vi "Set Focus Slider.vi"(8 "error in (no error)":errorcluster, 10 "Camera Parameter Information":T1, 11 "UI in":refnum<class "UI.lvclass">) -> (0 "error out":errorcluster)   [LabVIEW 2020, in "AR Example.lvlib" / "UI.lvclass"]
uses:
  UI.lvclass
  UI.lvclass/UI.ctl
  <vilib>/Utility/miscctls.llb/LVOutOfRangeActionTypeDef.ctl
  g_ar_toolkit.capture/Stream/Camera Parameter Information.ctl
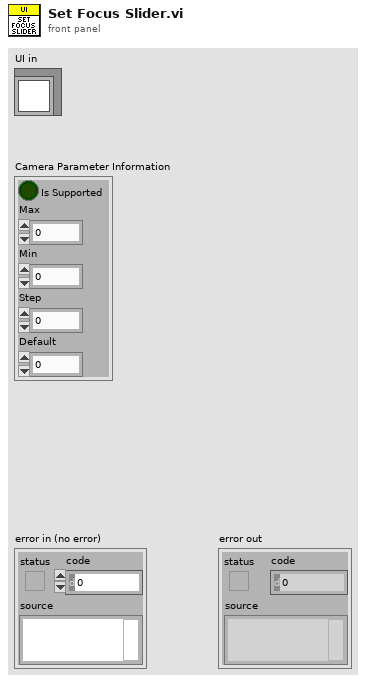
[diagram p1: front panel]
types:
  T1 = typedef "g_ar_toolkit.capture.lvlib/Stream.lvclass/Camera Parameter Information.ctl" = cluster{"Is Supported":bool, "Max":i32, "Min":i32, "Step":i32, "Default":i32}
  T2 = typedef "LVOutOfRangeActionTypeDef.ctl" = cluster{"Out of Range Action Minimum":u8, "Out of Range Action Maximum":u8, "Out of Range Action Increment":u8}
  T3 = enum8{"Enabled", "Disabled", "Disabled and Grayed Out"}
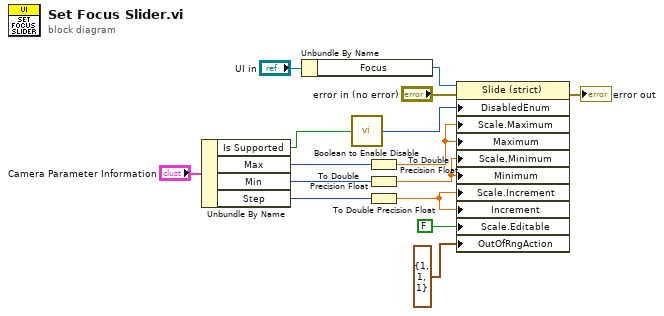
[diagram p0: block diagram]
diagram:
  n1 = Unbundle By Name("Camera Parameter Information") -> ("Is Supported"=w12:bool, "Max"=w6:i32, "Min"=w5:i32, "Step"=w4:i32)
  n2 = Unbundle By Name("UI in") -> ("Focus"=w14:refnum<vi>)
  n3 = call "Boolean to Enable Disable.vi"("Enable?"=w12) -> ("Enable/Disable"=w11:T3)
  n4 = To Double Precision Float(number=w6) -> (double precision float=w3:dbl)
  n5 = To Double Precision Float(number=w5) -> (double precision float=w2:dbl)
  n6 = To Double Precision Float(number=w4) -> (double precision float=w1:dbl)
  n7 = property class="Slide (strict)"(reference=w14, error in="error in (no error)", "DisabledEnum"=w11, "Scale.Maximum"=w3, "Maximum"=w3, "Scale.Minimum"=w2, "Minimum"=w2, "Scale.Increment"=w1, "Increment"=w1, "Scale.Editable"=FALSE, "OutOfRngAction"=T2 {"Out of Range Action Minimum"=1, "Out of Range Action Maximum"=1, "Out of Range Action Increment"=1} ("Response to Value Outside Limits")) -> (error out=→"error out":errorcluster)  [unwired: 1 out]
